vi "PCA BackProject.vi"(8 "error in (no error)":errorcluster, 9 "Result in":dbl[][](array[numeric]), 10 "Vectors":dbl[][](array[numeric]), 11 "PCA in":refnum<class "PCA.lvclass">) -> (0 "error out":errorcluster, 2 "Result out":dbl[][](array[numeric]), 3 "PCA out":refnum<class "PCA.lvclass">)   [LabVIEW 2020, in "OpenLvVision_OpenCv.lvlib" / "PCA.lvclass"]
doc: "Reconstructs vectors from their PC projections."
uses:
  PCA.lvclass
  C:/Users/lukas/Downloads/OpenLvVision_OpenCv/SourceCode/LabView/OpenLvVision_OpenCv/_LvHelpers/EdvrObject/EdvrObject.lvclass
  _LvHelpers/EdvrObject/EdvrObject.lvclass/EdvrObject.ctl
  _LvHelpers/MatHandling/WriteSize/WriteSizeMat_2DArray_DBL.vi
  _LvHelpers/MatHandling/RegisterMat/RegisterMat_Array2D-DBL.vi
  OpenLvVision_OpenCv.lvlib
  _LvHelpers/EdvrObject/EdvrObject.lvclass
  Dlls/OlvOpenCvWrapper.dll
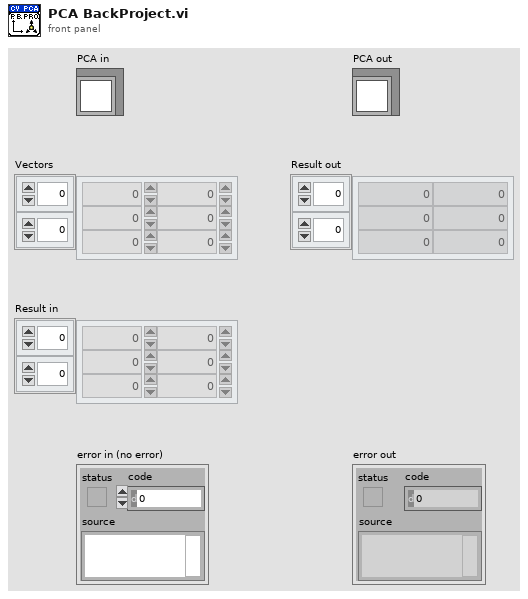
[diagram p1: front panel]
types:
  T1 = typedef "OpenLvVision_OpenCv.lvlib/MatInfo.ctl" = cluster{"Datatype":T2, "Height":i32, "Width":i32, "Channels":i32, "LineWidth":i32, "Null":u8}
  T2 = typedef "OpenLvVision_OpenCv.lvlib/LvDatatype.ctl" = enum32{"Undefined", "U8", "I8", "U16", "I16", "U32_Color", "I32", "U64_Color", "I64", "SGL", "DBL", "Complex SGL", "Complex DBL", "Array 1D U8", "Array 1D I8", "Array 1D U16", "Array 1D I16", "Array 1D U32_Color", "Array 1D I32", "Array 1D U64_Color", "Array 1D I64", "Array 1D SGL", "Array 1D DBL", "Array 1D Complex SGL", "Array 1D Complex DBL", "Array 2D U8", "Array 2D I8", "Array 2D U16", "Array 2D I16", "Array 2D U32", "Array 2D U32_Color", "Array 2D I32", "Array 2D U64", "Array 2D U64_Color", "Array 2D I64", "Array 2D SGL", "Array 2D DBL", "Array 2D Complex SGL", "Array 2D Complex DBL", "Image Mono U8", "Image Mono U16", "Image Mono I16", "Image Mono SGL", "Image Color U32", "Image Color U64", "ImageComplex Sgl", "Array1d_2dPointI32", "Array1d_2dPointSGL", "Array1d_2dPointDBL", "Array1d_3dPointI32", "Array1d_3dPointSGL", "Array1d_3dPointDBL", "Array1d_4dPointI32", "Array1d_4dPointSGL", "Array1d_4dPointDBL"}
  T3 = typedef "OpenLvVision_OpenCv.lvlib/EdvrObject.lvclass/Edvr.ctl" = refnum<data-value>
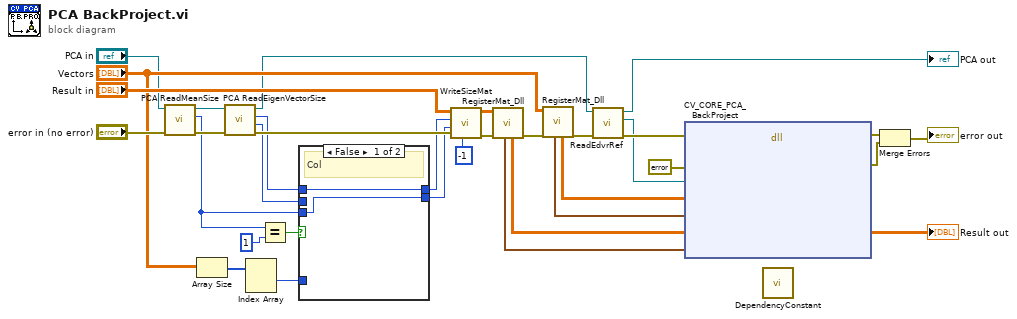
[diagram p0: block diagram]
diagram:
  n1 = call "PCA ReadMeanSize.vi"("error in (no error)"="error in (no error)", "PCA in"="PCA in") -> ("error out"=w14:errorcluster, "rows"=w1:i32, "PCA out"=w15:refnum<class "PCA.lvclass">)  [unwired: 6 in, 1 out]
  n2 = Array Size(array="Vectors") -> (size(s)=w6:i32[])
  n3 = call "PCA ReadEigenVectorSize.vi"("error in (no error)"=w14, "PCA in"=w15) -> ("error out"=w13:errorcluster, "cols"=w10:i32, "rows"=w11:i32, "PCA out"=w2:refnum<class "PCA.lvclass">)  [unwired: 6 in]
  n4 = Index Array(array=w6) -> (element #1=w5:i32)  [unwired: 2 in, 1 out]
  n5 = Equal?(x=w1, y=1) -> (x = y?=w12:bool)
  n6 = case shown="False" w12 {
    tunnel: w11 -> [w36 w38]
    tunnel: w10 -> [_ _]
    tunnel: [w36 w38] -> w9
    tunnel: w5 -> [_ w37]
    tunnel: [w35 w37] -> w4
    tunnel: w1 -> [w35 _]
    frame False {
      # "Col"
    }
    frame True {
      # "Row"
    }
  }
  n7 = call-poly "WriteSizeMat.vi"("Channel"=-1, "error in"=w13, "Height"=w4, "Width"=w9, "Array in"="Result in") -> ("error out"=w24:errorcluster, "Array out"=w25:dbl[][])  [unwired: 5 in]
  n8 = call-poly "RegisterMat_Dll.vi"("error in"=w24, "Array in"=w25) -> ("error out"=w22:errorcluster, "AdressOrData"=w20:dbl[][], "Mat"=w19:T1)  [unwired: 6 in, 1 out]
  n9 = call-poly "RegisterMat_Dll.vi"("error in"=w22, "Array in"="Vectors") -> ("error out"=w28:errorcluster, "AdressOrData"=w30:dbl[][], "Mat"=w29:T1)  [unwired: 6 in, 1 out]
  n10 = call "ReadEdvrRef.vi"("error in (no error)"=w28, "EdvrObject in"=w2) -> ("error out"=w27:errorcluster, "Edvr"=w26:T3, "EdvrObject out"=→"PCA out":refnum<class "PCA.lvclass">)  [unwired: 7 in]
  n11 = dll-call lib="C:/Users/lukas/Downloads/OpenLvVision_OpenCv/SourceCode/LabView/OpenLvVision_OpenCv/Dlls/OlvOpenCvWrapper.dll" fn="CV_CORE_PCA_BackProject"(error in=w27, "Error"=errorcluster {"status"=FALSE, "code"=0, "source"=""} ("error out"), "edvrRef"=w26, "addressData"=w30, "matInfoData"=w29, "addressResult"=w20, "matInfoResult"=w19) -> (error out=w32:errorcluster, "Error"=w31:errorcluster, "addressResult"=→"Result out":dbl[][])  [unwired: 7 in, 1 out]
  n12 = call "DependencyConstant.vi"() -> ()  [unwired: 12 in]
  n13 = Merge Errors(w32, w31) -> (→"error out":errorcluster)
